vi "Form Sentence.vi"(6 "error in (no error)":errorcluster, 8 "sentence data":string[](array[string]), 9 "sentence type":string) -> (0 "error out":errorcluster, 3 "sentence":string)   [LabVIEW 2017, in "NMEA API.lvlib"]
doc: "Creates an NMEA sentence formatted as the <B>sentence type</B> you specify and with the <B>sentence data</B> you specify. This VI also applies punctuation, a checksum, and termination characters to the sentence."
uses:
  <vilib>/robotics/Protocols/NMEA/NMEA API.lvlib
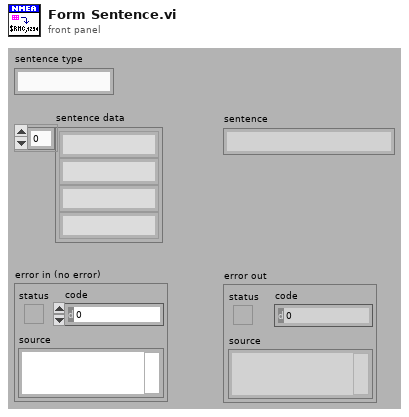
[diagram p1: front panel]
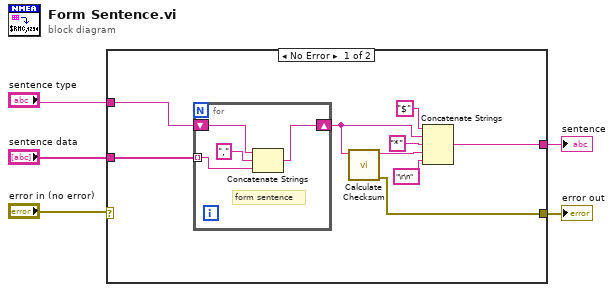
[diagram p0: block diagram]
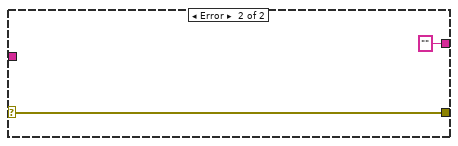
[diagram p2: hidden frame]
diagram:
  n1 = case shown="No Error" "error in (no error)" {
    selector: "error in (no error)" -> [_ w20]
    tunnel: [w9 w20] -> w4
    tunnel: [w8 ""] -> w3
    tunnel: "sentence type" -> [w7 _]
    tunnel: "sentence data" -> [w6 _]
    frame No Error {
      n2 = for {
        tunnel: w6 -> [w18] mode=indexing
        shift-right: [w17] -> w14
        shift-left: w7 -> [w16]
        # "form sentence"
        n3 = Concatenate Strings(w16, "," ("string"), w18) -> (w17:string)
      }
      n4 = call <vilib>:"Calculate Checksum.vi"("string"=w14) -> ("error out"=w9:errorcluster, "checksum"=w13:string)  [unwired: 7 in]
      n5 = Concatenate Strings("$" ("string"), w14, "*" ("string"), w13, "\r\n" ("string")) -> (w8:string)
    }
    frame Error {
    }
  }
  "error out" <- w4
  "sentence" <- w3
